vi "Close Right Slider.vi"(8 "error in (no error)":errorcluster, 11 "This VI":refnum<vi>) -> (0 "error out":errorcluster)   [LabVIEW 2014]
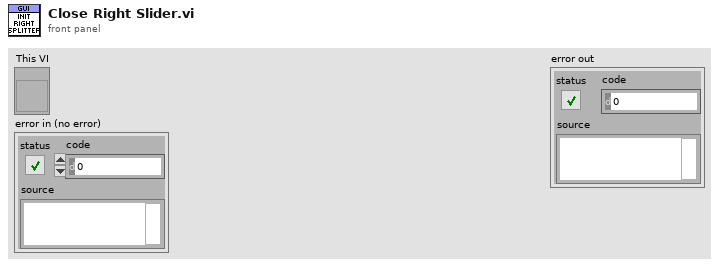
[diagram p1: front panel]
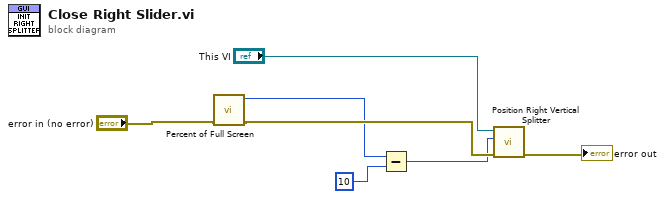
[diagram p0: block diagram]
diagram:
  n1 = call "Percent of Full Screen.vi"("error in (no error)"="error in (no error)") -> ("error out"=w4:errorcluster, "Right"=w3:i16)  [unwired: 8 in, 1 out]
  n2 = Subtract(x=w3, y=i16 10) -> (x-y=w1:i16)
  n3 = call "Position Right Vertical Splitter.vi"("error in (no error)"=w4, "Splitter Position"=w1, "This VI"="This VI") -> ("error out"=→"error out":errorcluster)  [unwired: 8 in]
